vi "Read Header Contents.vi"(8 "error in (no error)":errorcluster, 10 "String Header Contents":string, 11 "Construct String Header in":refnum<class "Construct String Header.lvclass">) -> (0 "error out":errorcluster, 2 "Header Contents":T1={"FILENAME"=["FILENAME", "example.fits", "File name at acquisition"], "OBSERVER"=["OBSERVER", "Denis", "Observer’s (PI) name"], "PROGRID"=["PROGRID", "2018A-001", "Program ID"], "OBJECT"=["OBJECT", "UNDEFINED", "Object name"], "NIGHTDIR"=["NIGHTDIR", "DIR", "Night directory name "], "CHANNEL"=["CHANNEL", "RED", "Instrument channel"], "INSTRUME"=["INSTRUME", "ECHARPE", "Instrument"], "NEXPSEQ"=["NEXPSEQ", "1", "Total number of exposures in sequence"], "SEQINDEX"=["SEQINDEX", "1", "Exposure index in the sequence"], "OBSTYPE"=["OBSTYPE", "BIAS", "Image type: OBJECT, BIAS, FLAT, ARC, DARK"], "READMOD"=["READMOD", "Normal", "Read out mode: fast, normal, slow"], "SHUTTER"=["SHUTTER", "CLOSED", "Shutter Mode (OPEN, CLOSED, or AUTO) "], "OPENSHT"=["OPENSHT", "50", "Time to open the shutter (ms) "], "CLOSESHT"=["CLOSESHT", "50", "Time to close the shutter (ms)"], "GAIN"=["GAIN", "3.38", "Gain (e-/ADU)"], "GAINERR "=["GAINERR", "0.05", " Gain error (e-/ADU)"], "RDNOISE"=["RDNOISE", "6.55", "Read noise (e-)"], "RNOISERR"=["RNOISERR", "0.02", "Read noise error (e-)"], "SKYFIBER"=["SKYFIBER", "\"OFF\"", "Sky fiber: ON or OFF"], "CALFIBER"=["CALFIBER", "\"OFF\"", "Calibration Fiber: ON or OFF"], "UTDATE"=["UTDATE", "'2017-10-01T20", "UT date at start of exposure"], "LOCTIME"=["LOCTIME", "'2017-10-01T17", "LT date at start of exposure"], "MJD"=["MJD", "58027.500000", "Modified Julian Date at start of exposure"], "OBSLON"=["OBSLON", "-45.57972", "Observatory East Longitude"], "OBSLAT"=["OBSLAT", "-22.53444", "Observatory Latitude"], "OBSALT"=["OBSALT", "1864.0", "Observatory elevation above sea level (m)"], "EXPTIME"=["EXPTIME", "1", "Exposure time (s)"], "TELRA"=["TELRA", "“00:00:00.000”", "TCS right ascension: “HH:MM:SS.SSS”"], "TELDEC"=["TELDEC", "“+00:00:00.000”", "TCS declination: “+-DD:MM:SS.SSS”"], "RA"=["RA", "“00:00:00.000”", "Requested right Ascension: “HH:MM:SS.SSS”"], "DEC"=["DEC", "“+00:00:00.000”", "Requested Declination: “+- DD:MM:SS.SSS”"], "RA_DEG"=["RA_DEG", "128.84946", "Requested Right Ascension (deg)"], "DEC_DEG"=["DEC_DEG", "+19.648717", "Requested Declination (deg)"], "EPOCH"=["EPOCH", "2000.00", "Epoch for Target coordinates"], "HA"=["HA", "“+01:13:05.98”", "Hour Angle (Sexagesimal)"], "HAD"=["HAD", "1.2183292", "Hour Angle (deg)"], "AIRMASS"=["AIRMASS", "1.085", "Mean airmass for the observation"], "AMSTART"=["AMSTART", "1.060", "Airmass at start of exposure"], "AMEND"=["AMEND", "1.114", "Airmass at end of exposure"], "XOFFSET"=["XOFFSET", "0.000000", "Telescope RA offset in arcsec"], "YOFFSET"=["YOFFSET", "0.000000", "Telescope DEC offset in arcsec"], "PA"=["PA", "14.6415392418", "Current Rotator Position Angle (degree)"], "CAMFOC"=["CAMFOC", "-3.53", "Camera focus position (mm)"], "TELFOC"=["TELFOC", "-3.53", "Telescope focus position (mm)"], "TCSUT"=["TCSUT", "‘23:17:24.8’", "TCS Universal Time"], "MOONDIST"=["MOONDIST", "60.0", "Moon angular distance to object (deg)"], "MOONALT"=["MOONALT", "15.0", "Moon elevation above horizon (deg)"], "MONNPHAS"=["MOONPHAS", "30.0", "Moon phase (deg)"], "ADC"=["ADC", "\"ON\"", "Atmospheric Dispersion Corrector: ON or OFF"], "ADCSPPED"=["ADCSPPED", "5.0", "ADC motor speed (rpm)"], "CALMIRR"=["CALMIRR", "\"OUT\"", "Calibration mirror position: IN or OUT"], "GUIDING"=["GUIDING", "“ON”", "Guider status: ON or OFF"], "GUIDTEXP"=["GUIDTEXP", "1.0", "Guider exposure time (s)"], "GUIDFREQ"=["GUIDFREQ", "1.0", "Guiding frequency (Hz)"], "GUIDOBJX"=["GUIDOBJX", "102.5", "Guiding object x position (pixel)"], "GUIDOBJY"=["GUIDOBJY", "300.3", "Guiding object y position (pixel)"], "AVGYCORR"=["AVGYCORR", "2.3", "Average correction in RA (arcsec)"], "AVGXCORR"=["AVGXCORR", "1.3", "Average correction in DEC (arcsec)"], "GFOCUS"=["GFOCUS", "3.0", "Guider focus position (mm)"], "THARLAMP"=["THARLAMP", "“OFF”", "Thorium-Argon lamp state: ON or OFF"], "HALLAMP"=["HALLAMP", "“OFF”", "Halogen lamp state: ON or OFF"], "AGITATOR"=["AGITATOR", "“ON”", "Fiber agitator: ON or OFF"], "THARMIRR"=["THARMIRR", "“SPECTROGRAPH”", "Th-Ar mirror position: SPECTROGRAPH or TELESCOPE"], "DSTATUS"=["DSTATUS", "‘OPEN’", "Dome Status: OPEN or CLOSED"], "DTEMP"=["DTEMP", "10.0", "Dome temperature (deg C)"], "DHUM"=["DHUM", "82.0", "Dome humidity (per cent)"], "DLAMP"=["DLAMP", "“OFF”", "Dome lamp: ON or OFF"], "DFLAT"=["DFLAT", "“OFF”", "Dome flat lamp: ON or OFF"], "TEMPEXT"=["TEMPEXT", "10.0", "External temperature (deg C)"], "PRESSURE"=["PRESSURE", "742.00", "Pressure (mbar)"], "HUMIDITY"=["HUMIDITY", "92.00", "Humidity (per cent)"], "WINDDIR"=["WINDDIR", "15.0", "Wind direction: North-eastward (deg)"], "WSPEED"=["WSPEED", "30.2", "Wind Speed (km/h)"], "TCSST"=["TCSST", "‘23:12:32.5’", "TCS Sideral Time"], "DPOS"=["DPOS", "0.00000", "Dome position (deg)"]}, 3 "Construct String Header out":refnum<class "Construct String Header.lvclass">)   [LabVIEW 2018, in "Construct String Header.lvclass"]
doc: "Este VI recebe uma string contendo as informações do header da imagem, retornando um cluster com as informações do header."
uses:
  Construct String Header.lvclass
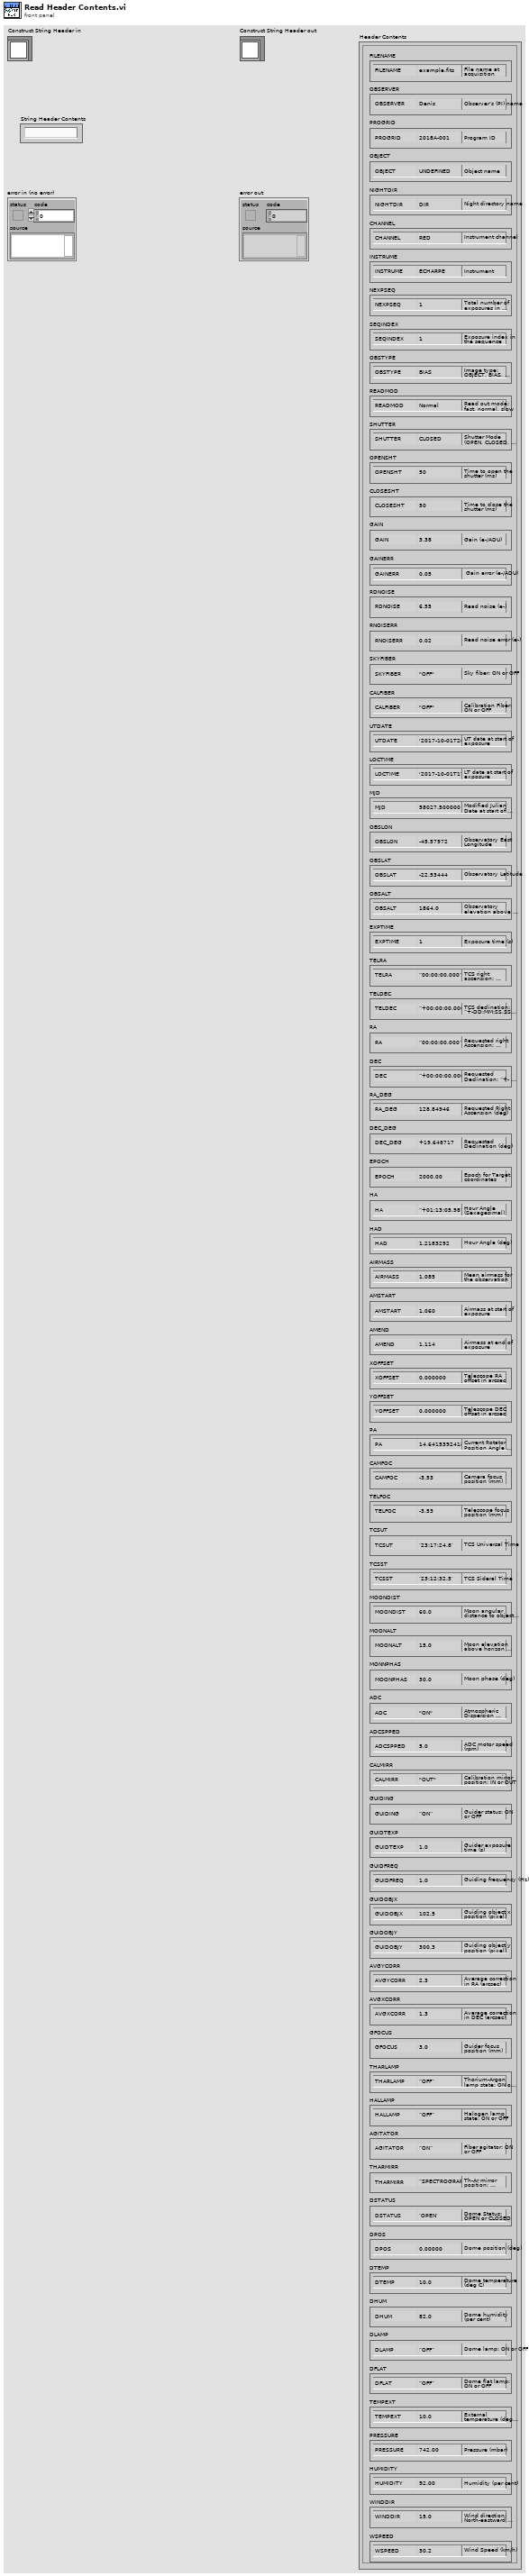
[diagram p1: front panel]
types:
  T1 = cluster{"FILENAME":string[], "OBSERVER":string[], "PROGRID":string[], "OBJECT":string[], "NIGHTDIR":string[], "CHANNEL":string[], "INSTRUME":string[], "NEXPSEQ":string[], "SEQINDEX":string[], "OBSTYPE":string[], "READMOD":string[], "SHUTTER":string[], "OPENSHT":string[], "CLOSESHT":string[], "GAIN":string[], "GAINERR ":string[], "RDNOISE":string[], "RNOISERR":string[], "SKYFIBER":string[], "CALFIBER":string[], "UTDATE":string[], "LOCTIME":string[], "MJD":string[], "OBSLON":string[], "OBSLAT":string[], "OBSALT":string[], "EXPTIME":string[], "TELRA":string[], "TELDEC":string[], "RA":string[], "DEC":string[], "RA_DEG":string[], "DEC_DEG":string[], "EPOCH":string[], "HA":string[], "HAD":string[], "AIRMASS":string[], "AMSTART":string[], "AMEND":string[], "XOFFSET":string[], "YOFFSET":string[], "PA":string[], "CAMFOC":string[], "TELFOC":string[], "TCSUT":string[], "MOONDIST":string[], "MOONALT":string[], "MONNPHAS":string[], "ADC":string[], "ADCSPPED":string[], "CALMIRR":string[], "GUIDING":string[], "GUIDTEXP":string[], "GUIDFREQ":string[], "GUIDOBJX":string[], "GUIDOBJY":string[], "AVGYCORR":string[], "AVGXCORR":string[], "GFOCUS":string[], "THARLAMP":string[], "HALLAMP":string[], "AGITATOR":string[], "THARMIRR":string[], "DSTATUS":string[], "DTEMP":string[], "DHUM":string[], "DLAMP":string[], "DFLAT":string[], "TEMPEXT":string[], "PRESSURE":string[], "HUMIDITY":string[], "WINDDIR":string[], "WSPEED":string[], "TCSST":string[], "DPOS":string[]}
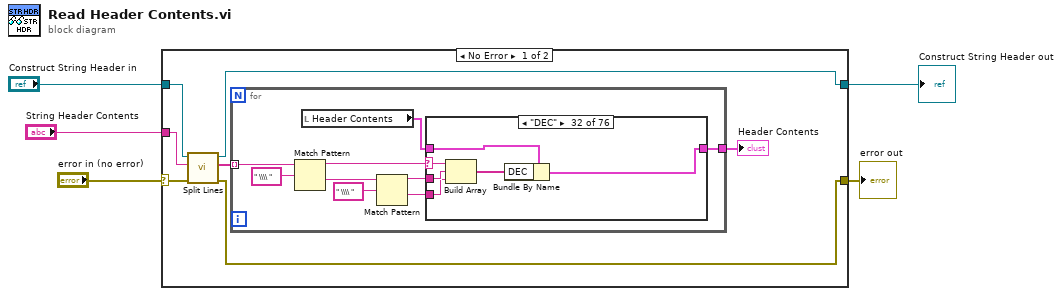
[diagram p0: block diagram]
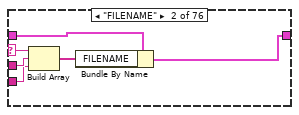
[diagram p3: hidden frame]
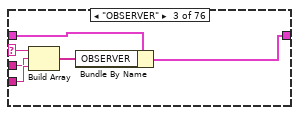
[diagram p4: hidden frame]
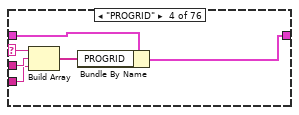
[diagram p5: hidden frame]
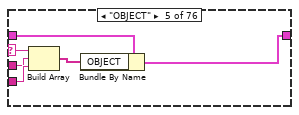
[diagram p6: hidden frame]
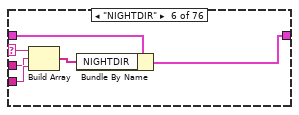
[diagram p7: hidden frame]
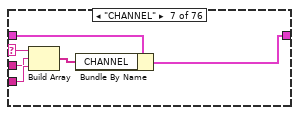
[diagram p8: hidden frame]
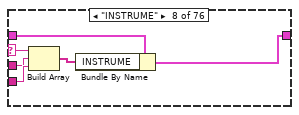
[diagram p9: hidden frame]
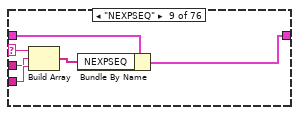
[diagram p10: hidden frame]
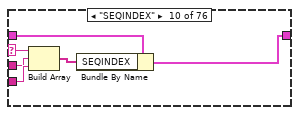
[diagram p11: hidden frame]
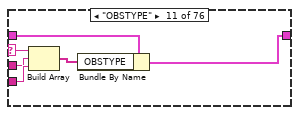
[diagram p12: hidden frame]
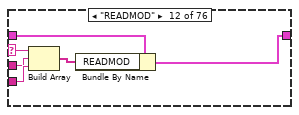
[diagram p13: hidden frame]
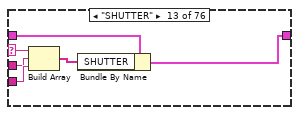
[diagram p14: hidden frame]
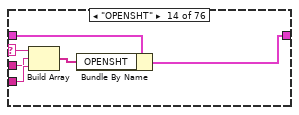
[diagram p15: hidden frame]
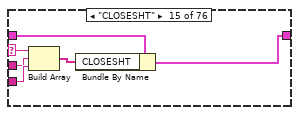
[diagram p16: hidden frame]
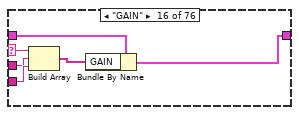
[diagram p17: hidden frame]
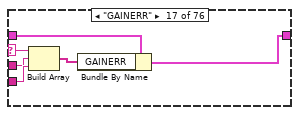
[diagram p18: hidden frame]
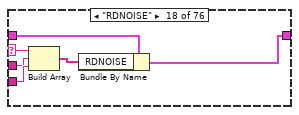
[diagram p19: hidden frame]
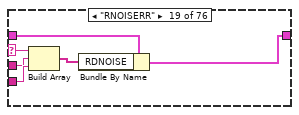
[diagram p20: hidden frame]
diagram:
  n1 = case shown="No Error" "error in (no error)" {
    selector: "error in (no error)" -> [w11 w473]
    tunnel: [w10 w473] -> w4
    tunnel: [w7 w474] -> w2
    tunnel: "Construct String Header in" -> [w12 w474]
    tunnel: "String Header Contents" -> [w9 _]
    frame No Error {
      n2 = call "Split Lines.vi"("error in (no error)"=w11, "spreadsheet string"=w9, "Construct String Header in"=w12) -> ("error out"=w10:errorcluster, "array"=w8:string[], "Construct String Header out"=w7:refnum<class "Construct String Header.lvclass">)  [unwired: 6 in]
      n3 = for {
        tunnel: w8 -> [w21] mode=indexing
        tunnel: [w14] -> w6
        n4 = Match Pattern(string=w21, regular expression=" \\\\ ") -> (before substring=w20:string, after substring=w18:string)  [unwired: 1 in, 2 out]
        n5 = local read "Header Contents"() -> (w13:T1)
        n6 = Match Pattern(string=w18, regular expression=" \\\\ ") -> (before substring=w16:string, after substring=w15:string)  [unwired: 1 in, 2 out]
        n7 = case shown="\"DEC\"" w20 {
          selector: w20 -> [_ w28 w30 w38 w42 w48 w54 w60 w66 w72 w78 w84 w90 w96 w102 w108 w114 w120 w126 w132 w138 w144 w150 w156 w162 w168 w174 w180 w186 w192 w198 w204 w210 w219 w222 w228 w234 w240 w246 w252 w258 w264 w270 w276 w282 w288 w294 w300 w306 w312 w318 w324 w330 w336 w342 w348 w354 w360 w366 w372 w378 w384 w390 w396 w402 w408 w414 w420 w426 w432 w441 w444 w450 w456 w462 w470]
          tunnel: [w22 w26 w33 w39 w46 w51 w57 w64 w70 w76 w81 w87 w93 w100 w105 w111 w117 w123 w129 w136 w141 w147 w154 w160 w166 w172 w177 w182 w190 w195 w200 w206 w213 w218 w226 w231 w238 w244 w249 w255 w261 w267 w274 w279 w285 w292 w298 w304 w310 w316 w321 w327 w333 w339 w346 w351 w357 w363 w370 w376 w382 w387 w393 w400 w405 w411 w418 w423 w429 w436 w440 w448 w453 w459 w466 w472] -> w14
          tunnel: w16 -> [_ w27 w31 w37 w43 w49 w55 w61 w67 w73 w79 w85 w91 w97 w103 w109 w115 w121 w127 w133 w139 w145 w151 w157 w163 w169 w175 w183 w187 w193 w201 w207 w211 w216 w223 w229 w235 w241 w247 w253 w259 w265 w271 w277 w283 w289 w295 w301 w307 w313 w319 w325 w331 w337 w343 w349 w355 w361 w367 w373 w379 w385 w391 w397 w403 w409 w415 w421 w427 w433 w438 w445 w451 w457 w463 w469]
          tunnel: w15 -> [_ w24 w32 w36 w44 w50 w56 w62 w68 w74 w80 w86 w92 w98 w104 w110 w116 w122 w128 w134 w140 w146 w152 w158 w164 w170 w176 w181 w188 w194 w199 w205 w212 w217 w224 w230 w236 w242 w248 w254 w260 w266 w272 w278 w284 w290 w296 w302 w308 w314 w320 w326 w332 w338 w344 w350 w356 w362 w368 w374 w380 w386 w392 w398 w404 w410 w416 w422 w428 w434 w439 w446 w452 w458 w464 w468]
          tunnel: w13 -> [w22 w23 w29 w35 w41 w47 w53 w59 w65 w71 w77 w83 w89 w95 w101 w107 w113 w119 w125 w131 w137 w143 w149 w155 w161 w167 w173 w179 w185 w191 w197 w203 w209 w215 w221 w227 w233 w239 w245 w251 w257 w263 w269 w275 w281 w287 w293 w299 w305 w311 w317 w323 w329 w335 w341 w347 w353 w359 w365 w371 w377 w383 w389 w395 w401 w407 w413 w419 w425 w431 w437 w443 w449 w455 w461 _]
          frame "False", Default {
          }
          frame "FILENAME" {
            n8 = Build Array(w28, w27, w24) -> (w25:string[])
            n9 = Bundle By Name(cluster=w23, "FILENAME"=w25) -> (w26:T1)
          }
          frame "OBSERVER" {
            n10 = Build Array(w30, w31, w32) -> (w34:string[])
            n11 = Bundle By Name(cluster=w29, "OBSERVER"=w34) -> (w33:T1)
          }
          frame "PROGRID" {
            n12 = Build Array(w38, w37, w36) -> (w40:string[])
            n13 = Bundle By Name(cluster=w35, "PROGRID"=w40) -> (w39:T1)
          }
          frame "OBJECT" {
            n14 = Build Array(w42, w43, w44) -> (w45:string[])
            n15 = Bundle By Name(cluster=w41, "OBJECT"=w45) -> (w46:T1)
          }
          frame "NIGHTDIR" {
            n16 = Build Array(w48, w49, w50) -> (w52:string[])
            n17 = Bundle By Name(cluster=w47, "NIGHTDIR"=w52) -> (w51:T1)
          }
          frame "CHANNEL" {
            n18 = Build Array(w54, w55, w56) -> (w58:string[])
            n19 = Bundle By Name(cluster=w53, "CHANNEL"=w58) -> (w57:T1)
          }
          frame "INSTRUME" {
            n20 = Build Array(w60, w61, w62) -> (w63:string[])
            n21 = Bundle By Name(cluster=w59, "INSTRUME"=w63) -> (w64:T1)
          }
          frame "NEXPSEQ" {
            n22 = Build Array(w66, w67, w68) -> (w69:string[])
            n23 = Bundle By Name(cluster=w65, "NEXPSEQ"=w69) -> (w70:T1)
          }
          frame "SEQINDEX" {
            n24 = Build Array(w72, w73, w74) -> (w75:string[])
            n25 = Bundle By Name(cluster=w71, "SEQINDEX"=w75) -> (w76:T1)
          }
          frame "OBSTYPE" {
            n26 = Build Array(w78, w79, w80) -> (w82:string[])
            n27 = Bundle By Name(cluster=w77, "OBSTYPE"=w82) -> (w81:T1)
          }
          frame "READMOD" {
            n28 = Build Array(w84, w85, w86) -> (w88:string[])
            n29 = Bundle By Name(cluster=w83, "READMOD"=w88) -> (w87:T1)
          }
          frame "SHUTTER" {
            n30 = Build Array(w90, w91, w92) -> (w94:string[])
            n31 = Bundle By Name(cluster=w89, "SHUTTER"=w94) -> (w93:T1)
          }
          frame "OPENSHT" {
            n32 = Build Array(w96, w97, w98) -> (w99:string[])
            n33 = Bundle By Name(cluster=w95, "OPENSHT"=w99) -> (w100:T1)
          }
          frame "CLOSESHT" {
            n34 = Build Array(w102, w103, w104) -> (w106:string[])
            n35 = Bundle By Name(cluster=w101, "CLOSESHT"=w106) -> (w105:T1)
          }
          frame "GAIN" {
            n36 = Build Array(w108, w109, w110) -> (w112:string[])
            n37 = Bundle By Name(cluster=w107, "GAIN"=w112) -> (w111:T1)
          }
          frame "GAINERR" {
            n38 = Build Array(w114, w115, w116) -> (w118:string[])
            n39 = Bundle By Name(cluster=w113, "GAINERR"=w118) -> (w117:T1)
          }
          frame "RDNOISE" {
            n40 = Build Array(w120, w121, w122) -> (w124:string[])
            n41 = Bundle By Name(cluster=w119, "RDNOISE"=w124) -> (w123:T1)
          }
          frame "RNOISERR" {
            n42 = Build Array(w126, w127, w128) -> (w130:string[])
            n43 = Bundle By Name(cluster=w125, "RDNOISE"=w130) -> (w129:T1)
          }
          frame "SKYFIBER" {
            n44 = Build Array(w132, w133, w134) -> (w135:string[])
            n45 = Bundle By Name(cluster=w131, "SKYFIBER"=w135) -> (w136:T1)
          }
          frame "CALFIBER" {
            n46 = Build Array(w138, w139, w140) -> (w142:string[])
            n47 = Bundle By Name(cluster=w137, "CALFIBER"=w142) -> (w141:T1)
          }
          frame "UTDATE" {
            n48 = Build Array(w144, w145, w146) -> (w148:string[])
            n49 = Bundle By Name(cluster=w143, "UTDATE"=w148) -> (w147:T1)
          }
          frame "LOCTIME" {
            n50 = Build Array(w150, w151, w152) -> (w153:string[])
            n51 = Bundle By Name(cluster=w149, "LOCTIME"=w153) -> (w154:T1)
          }
          frame "MJD" {
            n52 = Build Array(w156, w157, w158) -> (w159:string[])
            n53 = Bundle By Name(cluster=w155, "MJD"=w159) -> (w160:T1)
          }
          frame "OBSLON" {
            n54 = Build Array(w162, w163, w164) -> (w165:string[])
            n55 = Bundle By Name(cluster=w161, "OBSLON"=w165) -> (w166:T1)
          }
          frame "OBSLAT" {
            n56 = Build Array(w168, w169, w170) -> (w171:string[])
            n57 = Bundle By Name(cluster=w167, "OBSLAT"=w171) -> (w172:T1)
          }
          frame "OBSALT" {
            n58 = Build Array(w174, w175, w176) -> (w178:string[])
            n59 = Bundle By Name(cluster=w173, "OBSALT"=w178) -> (w177:T1)
          }
          frame "EXPTIME" {
            n60 = Build Array(w180, w183, w181) -> (w184:string[])
            n61 = Bundle By Name(cluster=w179, "EXPTIME"=w184) -> (w182:T1)
          }
          frame "TELRA" {
            n62 = Build Array(w186, w187, w188) -> (w189:string[])
            n63 = Bundle By Name(cluster=w185, "TELRA"=w189) -> (w190:T1)
          }
          frame "TELDEC" {
            n64 = Build Array(w192, w193, w194) -> (w196:string[])
            n65 = Bundle By Name(cluster=w191, "TELDEC"=w196) -> (w195:T1)
          }
          frame "RA" {
            n66 = Build Array(w198, w201, w199) -> (w202:string[])
            n67 = Bundle By Name(cluster=w197, "RA"=w202) -> (w200:T1)
          }
          frame "DEC" {
            n68 = Build Array(w204, w207, w205) -> (w208:string[])
            n69 = Bundle By Name(cluster=w203, "DEC"=w208) -> (w206:T1)
          }
          frame "RA_DEG" {
            n70 = Build Array(w210, w211, w212) -> (w214:string[])
            n71 = Bundle By Name(cluster=w209, "RA_DEG"=w214) -> (w213:T1)
          }
          frame "DEC_DEG" {
            n72 = Build Array(w219, w216, w217) -> (w220:string[])
            n73 = Bundle By Name(cluster=w215, "DEC_DEG"=w220) -> (w218:T1)
          }
          frame "EPOCH" {
            n74 = Build Array(w222, w223, w224) -> (w225:string[])
            n75 = Bundle By Name(cluster=w221, "EPOCH"=w225) -> (w226:T1)
          }
          frame "HA" {
            n76 = Build Array(w228, w229, w230) -> (w232:string[])
            n77 = Bundle By Name(cluster=w227, "HA"=w232) -> (w231:T1)
          }
          frame "HAD" {
            n78 = Build Array(w234, w235, w236) -> (w237:string[])
            n79 = Bundle By Name(cluster=w233, "HAD"=w237) -> (w238:T1)
          }
          frame "AIRMASS" {
            n80 = Build Array(w240, w241, w242) -> (w243:string[])
            n81 = Bundle By Name(cluster=w239, "AIRMASS"=w243) -> (w244:T1)
          }
          frame "AMSTART" {
            n82 = Build Array(w246, w247, w248) -> (w250:string[])
            n83 = Bundle By Name(cluster=w245, "AMSTART"=w250) -> (w249:T1)
          }
          frame "AMEND" {
            n84 = Build Array(w252, w253, w254) -> (w256:string[])
            n85 = Bundle By Name(cluster=w251, "AMEND"=w256) -> (w255:T1)
          }
          frame "XOFFSET" {
            n86 = Build Array(w258, w259, w260) -> (w262:string[])
            n87 = Bundle By Name(cluster=w257, "XOFFSET"=w262) -> (w261:T1)
          }
          frame "YOFFSET" {
            n88 = Build Array(w264, w265, w266) -> (w268:string[])
            n89 = Bundle By Name(cluster=w263, "YOFFSET"=w268) -> (w267:T1)
          }
          frame "PA" {
            n90 = Build Array(w270, w271, w272) -> (w273:string[])
            n91 = Bundle By Name(cluster=w269, "PA"=w273) -> (w274:T1)
          }
          frame "CAMFOC" {
            n92 = Build Array(w276, w277, w278) -> (w280:string[])
            n93 = Bundle By Name(cluster=w275, "CAMFOC"=w280) -> (w279:T1)
          }
          frame "TELFOC" {
            n94 = Build Array(w282, w283, w284) -> (w286:string[])
            n95 = Bundle By Name(cluster=w281, "TELFOC"=w286) -> (w285:T1)
          }
          frame "TCSUT" {
            n96 = Build Array(w288, w289, w290) -> (w291:string[])
            n97 = Bundle By Name(cluster=w287, "TCSUT"=w291) -> (w292:T1)
          }
          frame "MOONDIST" {
            n98 = Build Array(w294, w295, w296) -> (w297:string[])
            n99 = Bundle By Name(cluster=w293, "MOONDIST"=w297) -> (w298:T1)
          }
          frame "MOONALT" {
            n100 = Build Array(w300, w301, w302) -> (w303:string[])
            n101 = Bundle By Name(cluster=w299, "MOONALT"=w303) -> (w304:T1)
          }
          frame "MOONPHAS" {
            n102 = Build Array(w306, w307, w308) -> (w309:string[])
            n103 = Bundle By Name(cluster=w305, "MONNPHAS"=w309) -> (w310:T1)
          }
          frame "ADC" {
            n104 = Build Array(w312, w313, w314) -> (w315:string[])
            n105 = Bundle By Name(cluster=w311, "ADC"=w315) -> (w316:T1)
          }
          frame "ADCSPPED" {
            n106 = Build Array(w318, w319, w320) -> (w322:string[])
            n107 = Bundle By Name(cluster=w317, "ADCSPPED"=w322) -> (w321:T1)
          }
          frame "CALMIRR" {
            n108 = Build Array(w324, w325, w326) -> (w328:string[])
            n109 = Bundle By Name(cluster=w323, "CALMIRR"=w328) -> (w327:T1)
          }
          frame "GUIDING" {
            n110 = Build Array(w330, w331, w332) -> (w334:string[])
            n111 = Bundle By Name(cluster=w329, "GUIDING"=w334) -> (w333:T1)
          }
          frame "GUIDTEXP" {
            n112 = Build Array(w336, w337, w338) -> (w340:string[])
            n113 = Bundle By Name(cluster=w335, "GUIDTEXP"=w340) -> (w339:T1)
          }
          frame "GUIDFREQ" {
            n114 = Build Array(w342, w343, w344) -> (w345:string[])
            n115 = Bundle By Name(cluster=w341, "GUIDFREQ"=w345) -> (w346:T1)
          }
          frame "GUIDOBJX" {
            n116 = Build Array(w348, w349, w350) -> (w352:string[])
            n117 = Bundle By Name(cluster=w347, "GUIDOBJX"=w352) -> (w351:T1)
          }
          frame "GUIDOBJY" {
            n118 = Build Array(w354, w355, w356) -> (w358:string[])
            n119 = Bundle By Name(cluster=w353, "GUIDOBJY"=w358) -> (w357:T1)
          }
          frame "AVGYCORR" {
            n120 = Build Array(w360, w361, w362) -> (w364:string[])
            n121 = Bundle By Name(cluster=w359, "AVGYCORR"=w364) -> (w363:T1)
          }
          frame "AVGXCORR" {
            n122 = Build Array(w366, w367, w368) -> (w369:string[])
            n123 = Bundle By Name(cluster=w365, "AVGXCORR"=w369) -> (w370:T1)
          }
          frame "GFOCUS" {
            n124 = Build Array(w372, w373, w374) -> (w375:string[])
            n125 = Bundle By Name(cluster=w371, "GFOCUS"=w375) -> (w376:T1)
          }
          frame "THARLAMP" {
            n126 = Build Array(w378, w379, w380) -> (w381:string[])
            n127 = Bundle By Name(cluster=w377, "THARLAMP"=w381) -> (w382:T1)
          }
          frame "HALLAMP" {
            n128 = Build Array(w384, w385, w386) -> (w388:string[])
            n129 = Bundle By Name(cluster=w383, "HALLAMP"=w388) -> (w387:T1)
          }
          frame "AGITATOR" {
            n130 = Build Array(w390, w391, w392) -> (w394:string[])
            n131 = Bundle By Name(cluster=w389, "AGITATOR"=w394) -> (w393:T1)
          }
          frame "THARMIRR" {
            n132 = Build Array(w396, w397, w398) -> (w399:string[])
            n133 = Bundle By Name(cluster=w395, "THARMIRR"=w399) -> (w400:T1)
          }
          frame "DSTATUS" {
            n134 = Build Array(w402, w403, w404) -> (w406:string[])
            n135 = Bundle By Name(cluster=w401, "DSTATUS"=w406) -> (w405:T1)
          }
          frame "DTEMP" {
            n136 = Build Array(w408, w409, w410) -> (w412:string[])
            n137 = Bundle By Name(cluster=w407, "DTEMP"=w412) -> (w411:T1)
          }
          frame "DHUM" {
            n138 = Build Array(w414, w415, w416) -> (w417:string[])
            n139 = Bundle By Name(cluster=w413, "DHUM"=w417) -> (w418:T1)
          }
          frame "DLAMP" {
            n140 = Build Array(w420, w421, w422) -> (w424:string[])
            n141 = Bundle By Name(cluster=w419, "DLAMP"=w424) -> (w423:T1)
          }
          frame "DFLAT" {
            n142 = Build Array(w426, w427, w428) -> (w430:string[])
            n143 = Bundle By Name(cluster=w425, "DFLAT"=w430) -> (w429:T1)
          }
          frame "TEMPEXT" {
            n144 = Build Array(w432, w433, w434) -> (w435:string[])
            n145 = Bundle By Name(cluster=w431, "TEMPEXT"=w435) -> (w436:T1)
          }
          frame "PRESSURE" {
            n146 = Build Array(w441, w438, w439) -> (w442:string[])
            n147 = Bundle By Name(cluster=w437, "PRESSURE"=w442) -> (w440:T1)
          }
          frame "HUMIDITY" {
            n148 = Build Array(w444, w445, w446) -> (w447:string[])
            n149 = Bundle By Name(cluster=w443, "HUMIDITY"=w447) -> (w448:T1)
          }
          frame "WINDDIR" {
            n150 = Build Array(w450, w451, w452) -> (w454:string[])
            n151 = Bundle By Name(cluster=w449, "WINDDIR"=w454) -> (w453:T1)
          }
          frame "WSPEED" {
            n152 = Build Array(w456, w457, w458) -> (w460:string[])
            n153 = Bundle By Name(cluster=w455, "WSPEED"=w460) -> (w459:T1)
          }
          frame "TCSST" {
            n154 = Build Array(w462, w463, w464) -> (w465:string[])
            n155 = Bundle By Name(cluster=w461, "TCSST"=w465) -> (w466:T1)
          }
          frame "DPOS" {
            n156 = Build Array(w470, w469, w468) -> (w471:string[])
            n157 = local read "Header Contents"() -> (w467:T1)
            n158 = Bundle By Name(cluster=w467, "DPOS"=w471) -> (w472:T1)
          }
        }
      }
      "Header Contents" <- w6
    }
    frame Error {
    }
  }
  "error out" <- w4
  "Construct String Header out" <- w2
